vi "Varients creator data.vi"() -> ()   [LabVIEW 2017]
uses:
  <vilib>/Utility/config.llb/NI_LVConfig.lvlib
panel:
  out "Country":string[](array[string])
  out "data":T1
  in  "Varient Options":T1
  out "appended path":path
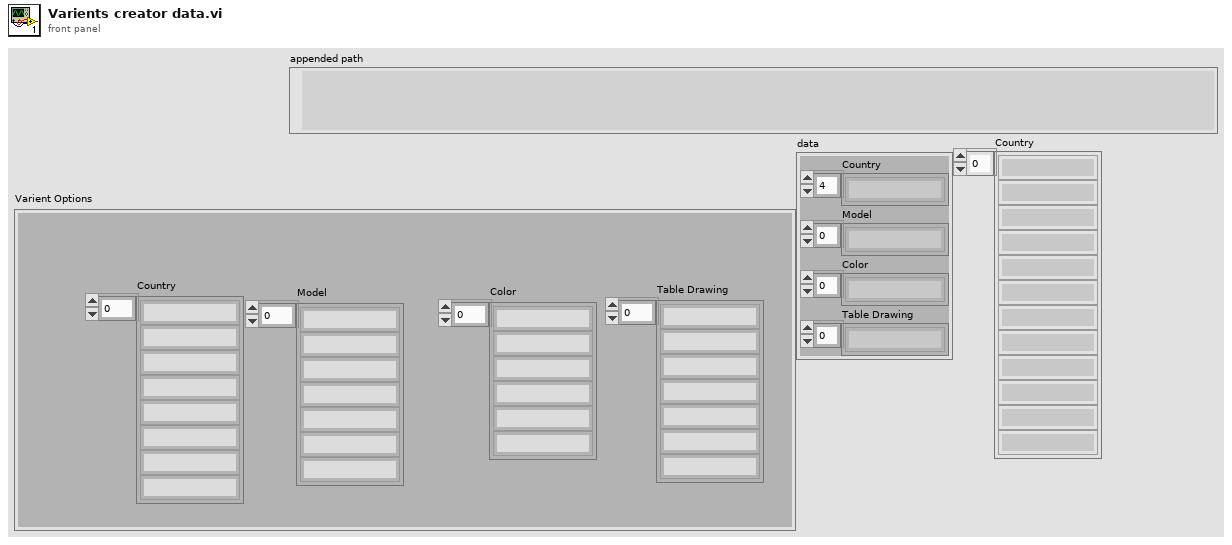
[diagram p1: front panel]
types:
  T1 = cluster{"Country":string[], "Model":string[], "Color":string[], "Table Drawing":string[]}
  T2 = enum32{"invalid app kind", "Development System", "Run Time System", "Student Edition", "Embedded LabVIEW", "Evaluation", "Custom"}
  T3 = typedef "NI_LVConfig.lvlib/Config Data RefNum.ctl" = refnum<k1>
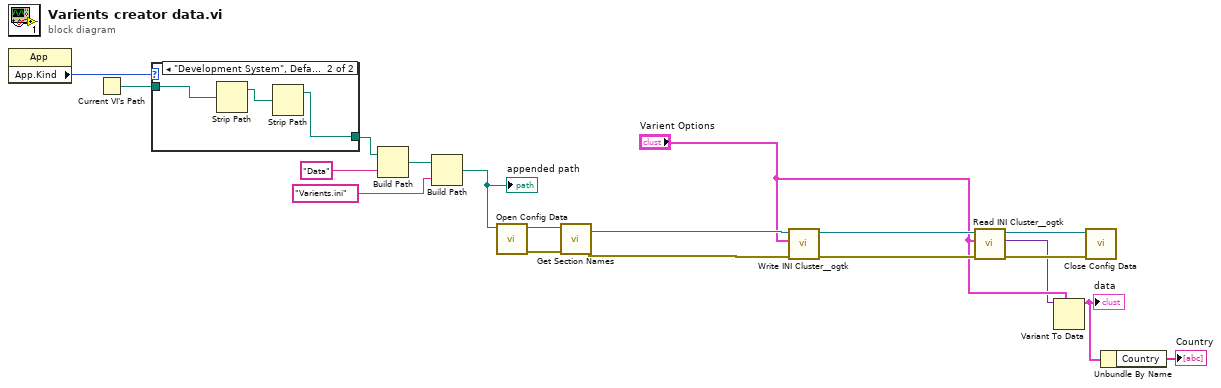
[diagram p0: block diagram]
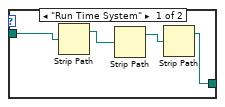
[diagram p2: hidden frame]
diagram:
  n1 = property class="App"() -> ("App.Kind"=w18:T2)  [unwired: 2 in, 2 out]
  n2 = Current VI's Path() -> (path=w19:path)
  n3 = case shown="\"Development System\", Default" w18 {
    tunnel: w19 -> [w21 w25]
    tunnel: [w20 w24] -> w12
    frame "Run Time System" {
      n4 = Strip Path(path=w21) -> (stripped path=w23:path)  [unwired: 1 out]
      n5 = Strip Path(path=w23) -> (stripped path=w22:path)  [unwired: 1 out]
      n6 = Strip Path(path=w22) -> (stripped path=w20:path)  [unwired: 1 out]
    }
    frame "Development System", Default {
      n7 = Strip Path(path=w25) -> (stripped path=w26:path)  [unwired: 1 out]
      n8 = Strip Path(path=w26) -> (stripped path=w24:path)  [unwired: 1 out]
    }
  }
  n9 = Build Path(base path=w12, name or relative path="Data") -> (appended path=w13:path)
  n10 = Build Path(base path=w13, name or relative path="Varients.ini") -> (appended path=w17:path)
  "appended path" <- w17
  n11 = call <vilib>:"Open Config Data.vi"("configuration file path"=w17) -> ("error out"=w11:errorcluster, "refnum"=w14:T3)  [unwired: 8 in, 1 out]
  n12 = call <vilib>:"Get Section Names.vi"("error in (no error)"=w11, "refnum"=w14) -> ("error out"=w9:errorcluster, "refnum out"=w10:T3)  [unwired: 7 in, 1 out]
  n13 = call <userlib>:"Write INI Cluster__ogtk.vi"("error in (no error)"=w9, "INI Fomatted Cluster"="Varient Options", "refnum"=w10) -> ("error out"=w6:errorcluster, "dup refnum"=w8:T3)  [unwired: 7 in]
  n14 = call <userlib>:"Read INI Cluster__ogtk.vi"("error in (no error)"=w6, "INI Fomatted Cluster Type"="Varient Options", "refnum"=w8) -> ("error out"=w5:errorcluster, "INI Fomatted Cluster"=w3:variant, "dup refnum"=w7:T3)  [unwired: 4 in, 2 out]
  n15 = Variant To Data(type="Varient Options", Variant=w3) -> (data=w2:T1)  [unwired: 1 in, 1 out]
  "data" <- w2
  n16 = call <vilib>:"Close Config Data.vi"("error in (no error)"=w5, "refnum"=w7) -> ()  [unwired: 8 in, 2 out]
  n17 = Unbundle By Name(w2) -> ("Country"=→"Country":string[])
